vi "Execution Unit.Async.vi"(10 "Parameters":variant, 11 "Process":refnum<class "Process.lvclass">) -> ()   [LabVIEW 2020, in "AIM ARINC 664 Engine.lvlib" / "Custom Device.lvlib"]
uses:
  Custom Device.lvlib
  <vilib>/NI/NIVS Inline Async API/_VS Inline Async API/Process/Process.lvclass
  Asynchronous Process Parameters.ctl
  Asynchronous Execution Unit Runtime Information.ctl
  Interfaces/Execution Unit/Execution Unit.lvclass
  Interfaces/Shared Resources/Shared Resources.lvclass
  <vilib>/NI/NIVS Inline Async API/_VS Inline Async API/Process/Process.lvclass/Process.ctl
  <vilib>/NI/NIVS Inline Async API/_Data Access Engine/Access Type Classes/ReadWrite/ReadWrite.lvclass/ReadWrite.ctl
  <vilib>/NI/NIVS Inline Async API/_Data Access Engine/Access Type Classes/Read/Read.lvclass/Read.ctl
  <vilib>/NI/NIVS Inline Async API/_Data Access Engine/Access Type Classes/Write/Write.lvclass/Write.ctl
  <vilib>/NI/NIVS Inline Async API/_Data Access Engine/Data Access Engine/Methods/Read.Data.vi
  <vilib>/NI/NIVS Inline Async API/_Data Access Engine/Data Access Engine/Methods/Write.Data.vi
  <vilib>/NI/NIVS Inline Async API/_Data Access Engine/Data Access Engine/Methods/ReadWrite.Data.vi
  <vilib>/NI/NIVS Inline Async API/_VS Inline Async API/Process/Data Member Access/Read Data Access.vi
  <vilib>/NI/NIVS Inline Async API/_VS Inline Async API/Error Handling Process/SubVIs/Error.ConvertArray.vi
  <vilib>/NI/NIVS Inline Async API/_Data Access Engine/Access Type Classes/Read/Read.ProcessData.vi
  <vilib>/NI/NIVS Inline Async API/_Data Access Engine/Access Type Classes/Write/Write.ProcessData.vi
  <vilib>/NI/NIVS Inline Async API/_Data Access Engine/Access Type Classes/ReadWrite/ReadWrite.ProcessData.vi
  <vilib>/NI/NIVS Inline Async API/_Data Access Engine/Access Type Classes/Write/Write.Buffer.vi
  <vilib>/NI/NIVS Inline Async API/_Data Access Engine/Access Type Classes/Write/Write.Commit.vi
  <vilib>/NI/NIVS Inline Async API/_Data Access Engine/Data Access Engine/Methods/Write.Lookup.vi
  <vilib>/NI/NIVS Inline Async API/_Data Access Engine/Data Access Engine/Methods/ReadWrite.Lookup.vi
  <vilib>/NI/NIVS Inline Async API/_Data Access Engine/Data Access Engine/Methods/Read.Lookup.vi
  <vilib>/NI/NIVS Inline Async API/_Data Access Engine/Data Access Engine/Data Access Engine.lvclass
  <vilib>/NI/NIVS Inline Async API/_Data Access Engine/Access Type Classes/ReadWrite/ReadWrite.lvclass
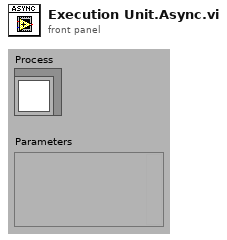
[diagram p1: front panel]
types:
  T1 = typedef "AIM ARINC 664 Engine.lvlib/Custom Device.lvlib/Asynchronous Process Parameters.ctl" = cluster{"Asynchronous Execution Unit Runtime Information":T2, "shared resources":refnum<class "Shared Resources.lvclass">}
  T2 = typedef "AIM ARINC 664 Engine.lvlib/Custom Device.lvlib/Asynchronous Execution Unit Runtime Information.ctl" = cluster{"Execution Unit":refnum<class "Execution Unit.lvclass">, "Incoming Channel Group Name":string, "Outgoing Channel Group Name":string, "ReadWrite Channel Group Name":string}
  T3 = typedef "Data Access Engine.lvlib/Data Access Engine.lvclass/Write.DVR.ctl" = refnum<data-value>
  T4 = typedef "Data Access Engine.lvlib/Data Access Engine.lvclass/ReadWrite.DVR.ctl" = refnum<data-value>
  T5 = typedef "Data Access Engine.lvlib/Data Access Engine.lvclass/Read.DVR.ctl" = refnum<data-value>
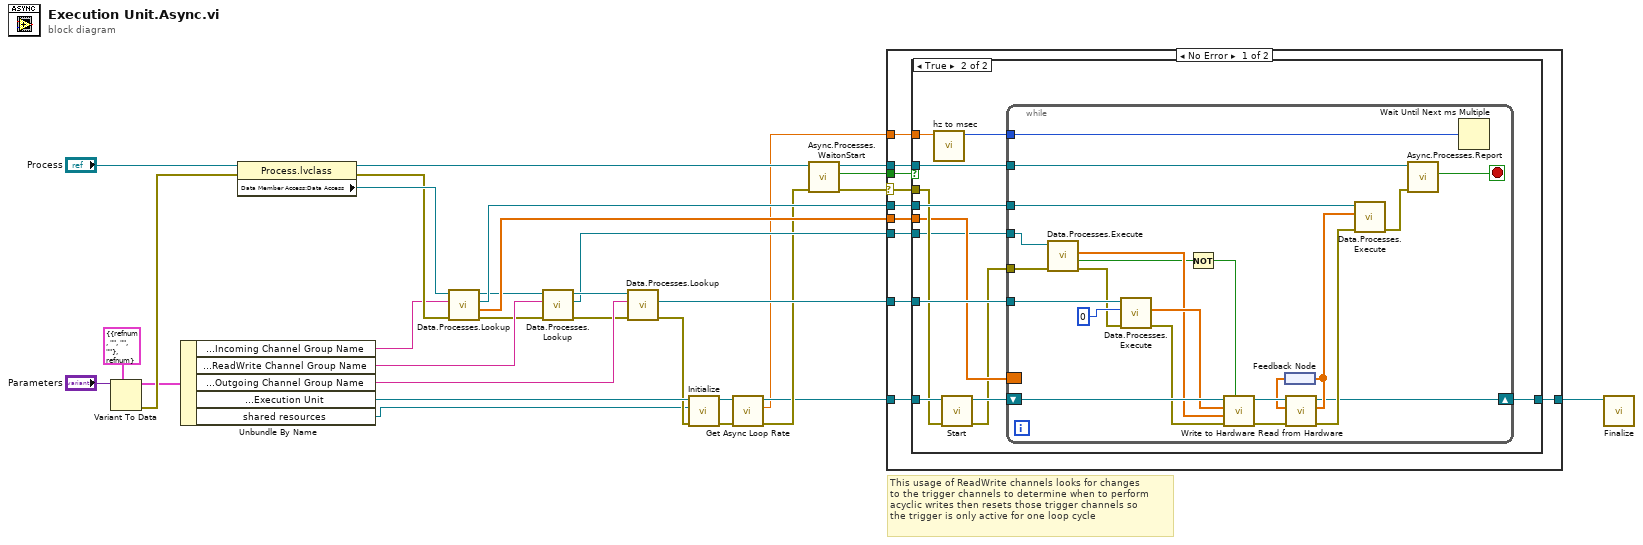
[diagram p0: block diagram]
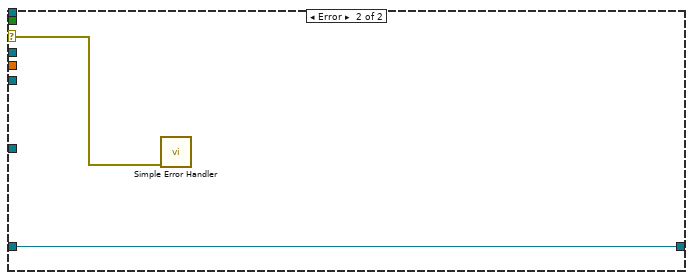
[diagram p3: hidden frame]
diagram:
  # "This usage of ReadWrite channels looks for changes\nto the trigger channels to determine when to perform\nacyclic writes then resets those trigger channels so\nthe trigger is only active for one loop cycle"
  n1 = Variant To Data(type=T1 {"Asynchronous Execution Unit Runtime Information"={"Execution Unit"=refnum, "Incoming Channel Group Name"="", "Outgoing Channel Group Name"="", "ReadWrite Channel Group Name"=""}, "shared resources"=refnum} ("Asynchronous Process Parameters"), Variant="Parameters") -> (data=w19:T1, error out=w20:errorcluster)  [unwired: 1 in]
  n2 = Unbundle By Name(w19) -> ("Asynchronous Execution Unit Runtime Information.Incoming Channel Group Name"=w12:string, "Asynchronous Execution Unit Runtime Information.ReadWrite Channel Group Name"=w11:string, "Asynchronous Execution Unit Runtime Information.Outgoing Channel Group Name"=w18:string, "Asynchronous Execution Unit Runtime Information.Execution Unit"=w16:refnum<class "Execution Unit.lvclass">, "shared resources"=w13:refnum<class "Shared Resources.lvclass">)
  n3 = property class="Process.lvclass"(reference="Process", error in=w20) -> (reference out=w25:refnum<class "Process.lvclass">, error out=w23:errorcluster, "Data Member Access:Data Access"=w24:refnum<class "Data Access Engine.lvclass">)
  n4 = call-poly <vilib>:"Data.Processes.Lookup.vi"("error in (no error)"=w23, "Name"=w12, "Data Access API in"=w24) -> ("error out"=w7:errorcluster, "Initial Values"=w17:dbl[], "Ref"=w27:T3, "Data Access API out"=w10:refnum<class "Data Access Engine.lvclass">)  [unwired: 5 in]
  n5 = call-poly <vilib>:"Data.Processes.Lookup.vi"("error in (no error)"=w7, "Name"=w11, "Data Access API in"=w10) -> ("error out"=w6:errorcluster, "Ref"=w8:T4, "Data Access API out"=w9:refnum<class "Data Access Engine.lvclass">)  [unwired: 5 in, 1 out]
  n6 = call-poly <vilib>:"Data.Processes.Lookup.vi"("error in (no error)"=w6, "Name"=w18, "Data Access API in"=w9) -> ("error out"=w15:errorcluster, "Ref"=w28:T5)  [unwired: 5 in, 2 out]
  n7 = call-dynamic "Initialize.vi"("error in (no error)"=w15, "shared resources"=w13, "Execution Unit in"=w16) -> ("error out"=w4:errorcluster, "Execution Unit out"=w5:refnum<class "Execution Unit.lvclass">)  [unwired: 7 in]
  n8 = call-dynamic "Get Async Loop Rate.vi"("error in (no error)"=w4, "Execution Unit in"=w5) -> ("error out"=w3:errorcluster, "Loop Rate Hz"=w1:dbl, "Execution Unit out"=w2:refnum<class "Execution Unit.lvclass">)  [unwired: 7 in]
  n9 = call <vilib>:"Async.Processes.WaitonStart.vi"("error in (no error)"=w3, "Process"=w25) -> ("error out"=w29:errorcluster, "Execute"=w31:bool, "Process out"=w30:refnum<class "Process.lvclass">)  [unwired: 7 in]
  n10 = case shown="No Error" w29 {
    selector: w29 -> [w37 w78]
    tunnel: w31 -> [w41 _]
    tunnel: w30 -> [w40 _]
    tunnel: w27 -> [w39 _]
    tunnel: w28 -> [w38 _]
    tunnel: w17 -> [w36 _]
    tunnel: w2 -> [w35 w77]
    tunnel: [w34 w77] -> w14
    tunnel: w8 -> [w33 _]
    tunnel: w1 -> [w32 _]
    frame No Error {
      n11 = case shown="True" w41 {
        tunnel: w37 -> [_ w50]
        tunnel: w40 -> [_ w52]
        tunnel: w38 -> [_ w54]
        tunnel: w39 -> [_ w53]
        tunnel: w36 -> [_ w48]
        tunnel: w35 -> [w42 w51]
        tunnel: [w42 w47] -> w34
        tunnel: w33 -> [_ w46]
        tunnel: w32 -> [_ w44]
        frame False {
        }
        frame True {
          n12 = call "hz to msec.vi"("Loop Rate Hz"=w44) -> ("msec"=w43:u32)  [unwired: 10 in]
          n13 = call-dynamic "Start.vi"("error in (no error)"=w50, "Execution Unit in"=w51) -> ("error out"=w45:errorcluster, "Execution Unit out"=w49:refnum<class "Execution Unit.lvclass">)  [unwired: 8 in]
          n14 = while {
            tunnel: w52 -> [w76]
            tunnel: w54 -> [w74]
            tunnel: w53 -> [w73]
            border: w48 -> [_]
            shift-right: [w63] -> w47
            shift-left: w49 -> [w71]
            tunnel: w46 -> [w62]
            tunnel: w45 -> [w61]
            tunnel: w43 -> [w55]
            stop <- w75 stop-if-true
            n15 = call-poly <vilib>:"Data.Processes.Execute.vi"("error in (no error)"=w61, "Ref"=w62) -> ("error out"=w59:errorcluster, "Timeout?"=w58:bool, "Data"=w60:dbl[])  [unwired: 6 in, 1 out]
            n16 = call-poly <vilib>:"Data.Processes.Execute.vi"("error in (no error)"=w59, "timeout ms"=0, "Ref"=w74) -> ("error out"=w68:errorcluster, "Values"=w69:dbl[])  [unwired: 6 in, 1 out]
            n17 = Not(x=w58) -> (.not. x?=w57:bool)
            n18 = call-dynamic "Write to Hardware.vi"("Valid Triggers"=w57, "error in (no error)"=w68, "Trigger Values"=w60, "Values in"=w69, "Execution Unit in"=w71) -> ("error out"=w56:errorcluster, "Execution Unit out"=w70:refnum<class "Execution Unit.lvclass">)  [unwired: 3 in, 2 out]
            n19 = feedback #1() -> (w65:dbl[])
            n20 = call-dynamic "Read from Hardware.vi"("error in (no error)"=w56, "Values in"=w65, "Execution Unit in"=w70) -> ("error out"=w67:errorcluster, "Values out"=w64:dbl[], "Execution Unit out"=w63:refnum<class "Execution Unit.lvclass">)  [unwired: 6 in]
            n21 = feedback-in #1(w64) -> ()
            n22 = call-poly <vilib>:"Data.Processes.Execute.vi"("error in (no error)"=w67, "Values"=w64, "Ref"=w73) -> ("error out"=w66:errorcluster)  [unwired: 8 in]
            n23 = call <vilib>:"Async.Processes.Report.vi"("Error"=w66, "Process in"=w76) -> ("Stop"=w75:bool)  [unwired: 8 in, 1 out]
            n24 = Wait Until Next ms Multiple(millisecond multiple=w55) -> ()  [unwired: 1 out]
          }
        }
      }
    }
    frame Error {
      n25 = call <vilib>:"Simple Error Handler.vi"("error in (no error)"=w78) -> ()  [unwired: 4 in, 5 out]
    }
  }
  n26 = call-dynamic "Finalize.vi"("Execution Unit in"=w14) -> ()  [unwired: 9 in, 2 out]
